vi "GetM1M3SupportEvents.vi"(8 "error in (no error)":errorcluster, 11 "Model in":refnum<class "Model.lvclass">) -> (0 "error out":errorcluster, 2 "M1M3 Support Events out":refnum<class "M1M3 Support Events.lvclass">, 3 "Model out":refnum<class "Model.lvclass">)   [LabVIEW 2016, in "Model.lvclass"]
uses:
  Model.lvclass
  M1M3 Support Events/M1M3 Support Events.lvclass
  Model.lvclass/Model.ctl
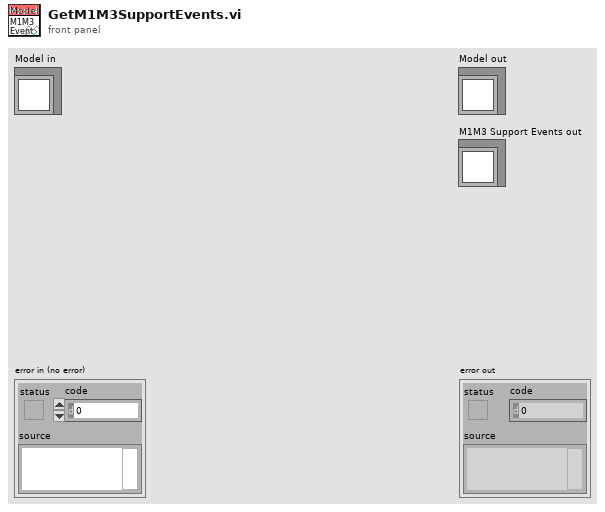
[diagram p1: front panel]
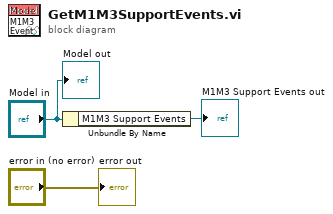
[diagram p0: block diagram]
diagram:
  n1 = Unbundle By Name("Model in") -> ("M1M3 Support Events"=→"M1M3 Support Events out":refnum<class "M1M3 Support Events.lvclass">)
  "error out" <- "error in (no error)"
  "Model out" <- "Model in"
